vi "First_Light.vi"() -> ()   [LabVIEW 2026]
uses:
  <vilib>/measure/NI_MABase.lvlib
panel:
  in  "stop":bool
  in  "Amplitude":dbl
  out "Waveform Chart":dynamicdata(graph)
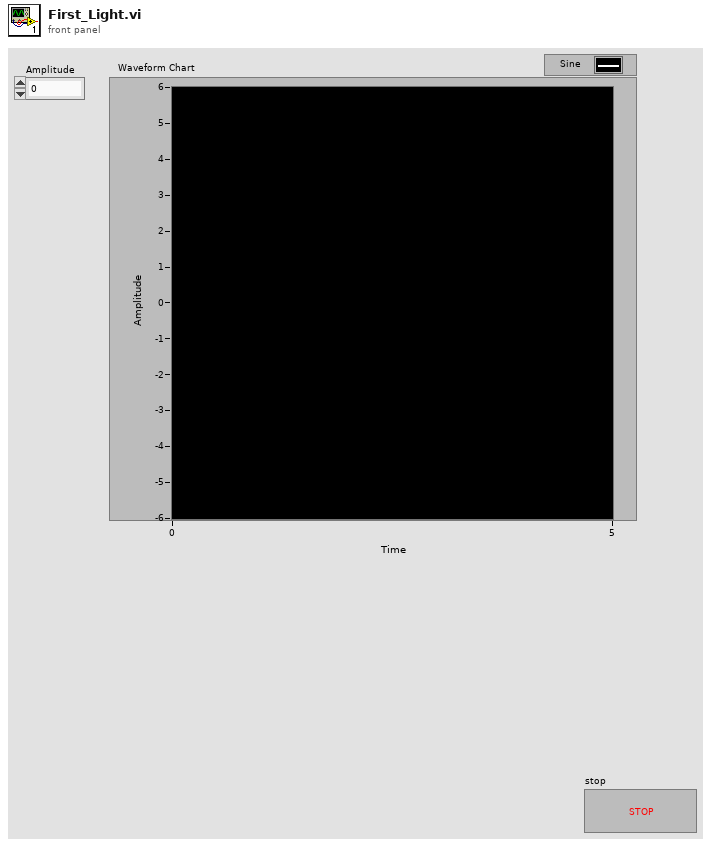
[diagram p1: front panel]
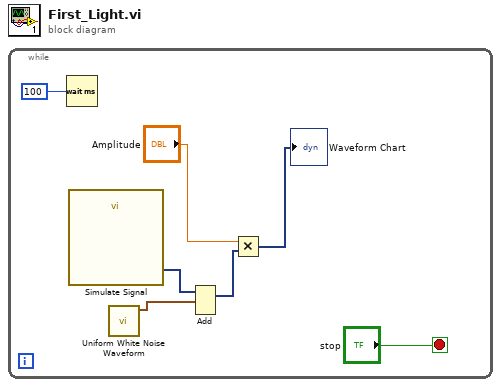
[diagram p0: block diagram]
diagram:
  n1 = while {
    stop <- "stop" stop-if-true
    n2 = Wait (ms)(milliseconds to wait=u32 100) -> ()  [unwired: 1 out]
    n3 = call "Simulate Signal"() -> ("Sine"=w5:dynamicdata)  [unwired: 14 in, 1 out]
    n4 = call <vilib>:"Uniform White Noise Waveform.vi"() -> ("signal out"=w4:waveform(dbl))  [unwired: 10 in, 1 out]
    n5 = Add(1:w4, 2:w5) -> (0:w3:dynamicdata)  [unwired: 1 in, 1 out]
    n6 = Multiply(x="Amplitude", y=w3) -> (x*y=→"Waveform Chart":dynamicdata)
  }
